vi "read config ini data.vi"(8 "error in (no error)":errorcluster, 11 "Refnum in":T1) -> (0 "error out":errorcluster, 2 "data out":T2, 3 "Refnum out":T1)   [LabVIEW 2024, in "Config Files Management.lvlib"]
doc: "This function reads the complete data from a configuration .ini file and stores it in an output cluster. The output cluster contains three string arrays: a 2-D array for the sections, where the first row stores the section names and the second row contains the number of keys in each section; a 1-D string array for the key names; and a 1-D string array for the corresponding values."
uses:
  Config Files Management.lvlib
  <vilib>/Utility/config.llb/NI_LVConfig.lvlib
  <vilib>/Utility/config.llb/Read Key (String).vi
  config data--cluster.ctl
  <vilib>/Utility/config.llb/Config Data RefNum.ctl
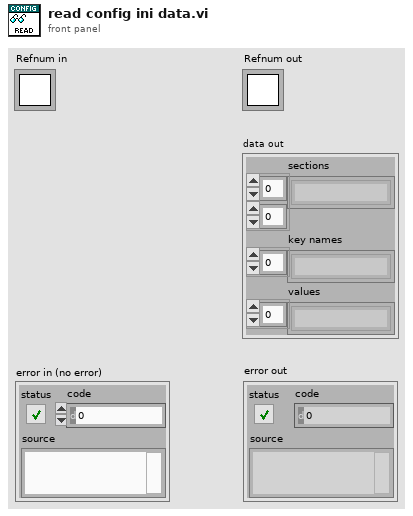
[diagram p1: front panel]
types:
  T1 = typedef "NI_LVConfig.lvlib/Config Data RefNum.ctl" = refnum<k1>
  T2 = typedef "Config Files Management.lvlib/config data--cluster.ctl" = cluster{"sections":string[][], "key names":string[], "values":string[]}
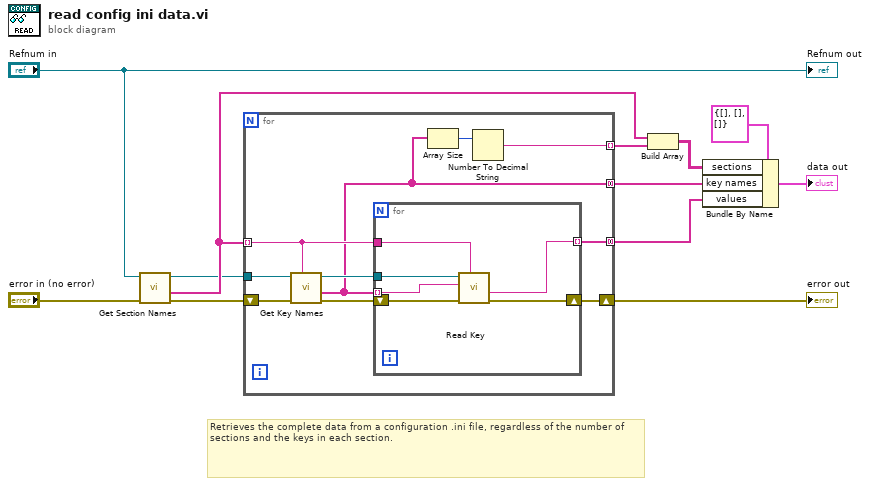
[diagram p0: block diagram]
diagram:
  # "Retrieves the complete data from a configuration .ini file, regardless of the number of sections and the keys in each section."
  n1 = call <vilib>:"Get Section Names.vi"("error in (no error)"="error in (no error)", "refnum"="Refnum in") -> ("error out"=w5:errorcluster, "section names"=w10:string[], "refnum out"=w4:T1)  [unwired: 7 in]
  n2 = for {
    shift-right: [w18] -> w2
    shift-left: w5 -> [w21]
    tunnel: w4 -> [w22]
    tunnel: w10 -> [w16] mode=indexing
    tunnel: [w15] -> w12 mode=concatenating
    tunnel: [w17] -> w11 mode=concatenating
    tunnel: [w13] -> w9 mode=indexing
    n3 = call <vilib>:"Get Key Names.vi"("section"=w16, "error in (no error)"=w21, "refnum"=w22) -> ("error out"=w20:errorcluster, "key names"=w15:string[], "refnum out"=w19:T1)  [unwired: 5 in, 1 out]
    n4 = for {
      shift-right: [w23] -> w18
      shift-left: w20 -> [w28]
      tunnel: w15 -> [w24] mode=indexing
      tunnel: w19 -> [w27]
      tunnel: w16 -> [w26]
      tunnel: [w25] -> w17 mode=indexing
      n5 = call-poly <vilib>:"Read Key.vi"("section"=w26, "error in (no error)"=w28, "key"=w24, "refnum"=w27) -> ("error out"=w23:errorcluster, "value"=w25:string)  [unwired: 4 in, 2 out]
    }
    n6 = Array Size(array=w15) -> (size(s)=w14:i32)
    n7 = Number To Decimal String(number=w14) -> (decimal integer string=w13:string)  [unwired: 1 in]
  }
  "error out" <- w2
  n8 = Build Array(w10, w9) -> (w8:string[][])
  n9 = Bundle By Name(cluster=T2 {"sections"=[], "key names"=[], "values"=[]} ("user data out"), "sections"=w8, "key names"=w12, "values"=w11) -> (→"data out":T2)
  "Refnum out" <- "Refnum in"
